vi "exercise6_error.vi"() -> ()   [LabVIEW 2018]
uses:
  <vilib>/Waveform/WDTFileIO.llb/Export Waveforms to Spreadsheet File.vi
  <vilib>/measure/NI_MABase.lvlib
panel:
  in  "amplitude":dbl=1.0 format="%0.2p"
  in  "frequency":dbl=10.0 format="%0.2p"
  out "Waveform Graph":waveform(dbl)[](graph)
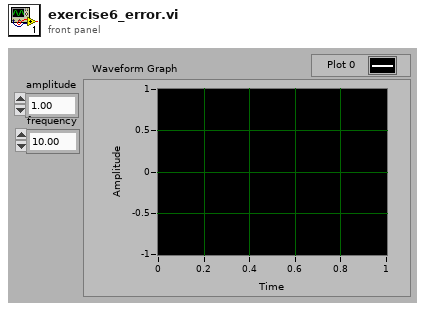
[diagram p1: front panel]
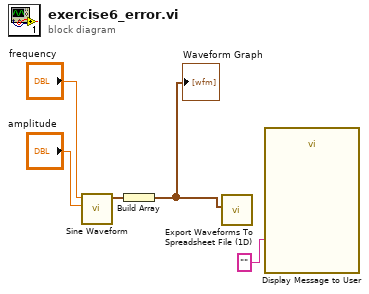
[diagram p0: block diagram]
diagram:
  n1 = call <vilib>:"Sine Waveform.vi"("amplitude"="amplitude", "frequency"="frequency") -> ("signal out"=w2:waveform(dbl))  [unwired: 8 in, 1 out]
  n2 = Build Array(w2) -> (w1:waveform(dbl)[])
  "Waveform Graph" <- w1
  n3 = call-poly <vilib>:"Export Waveforms To Spreadsheet File (1D).vi"("waveforms"=w1) -> ()  [unwired: 9 in, 2 out]
  n4 = call "Display Message to User"("Message"="") -> ()  [unwired: 9 in, 2 out]
